vi "Day 9 Task 1 attempt 2.vi"() -> ()   [LabVIEW 2018]
panel:
  out "sum":i32
  out "x+1":i32[][](array[numeric])
  out "subarray":bool[][](array[boolean])
  out "appended array":i32[][](array[numeric])
  out "Array":bool[][](array[boolean])
  out "logical AND":bool
  out "Original Array":i32[][](array[numeric])
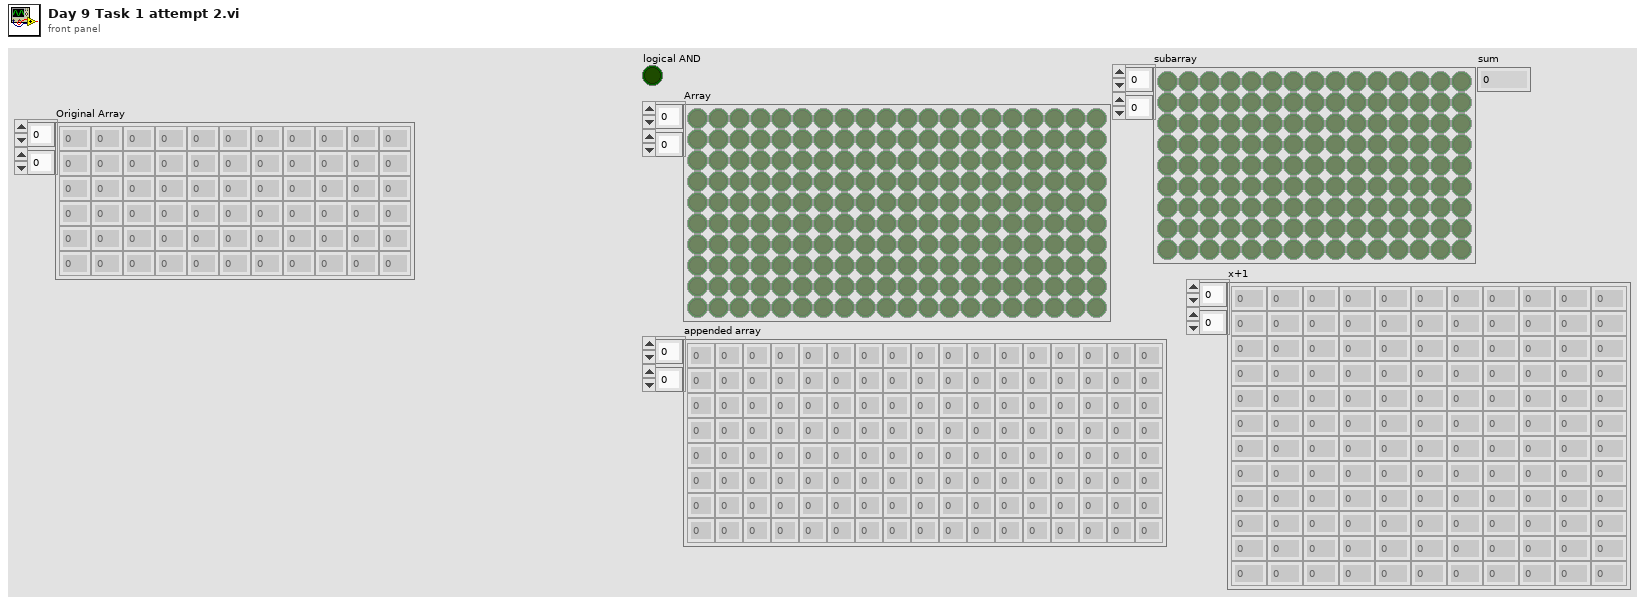
[diagram p1: front panel]
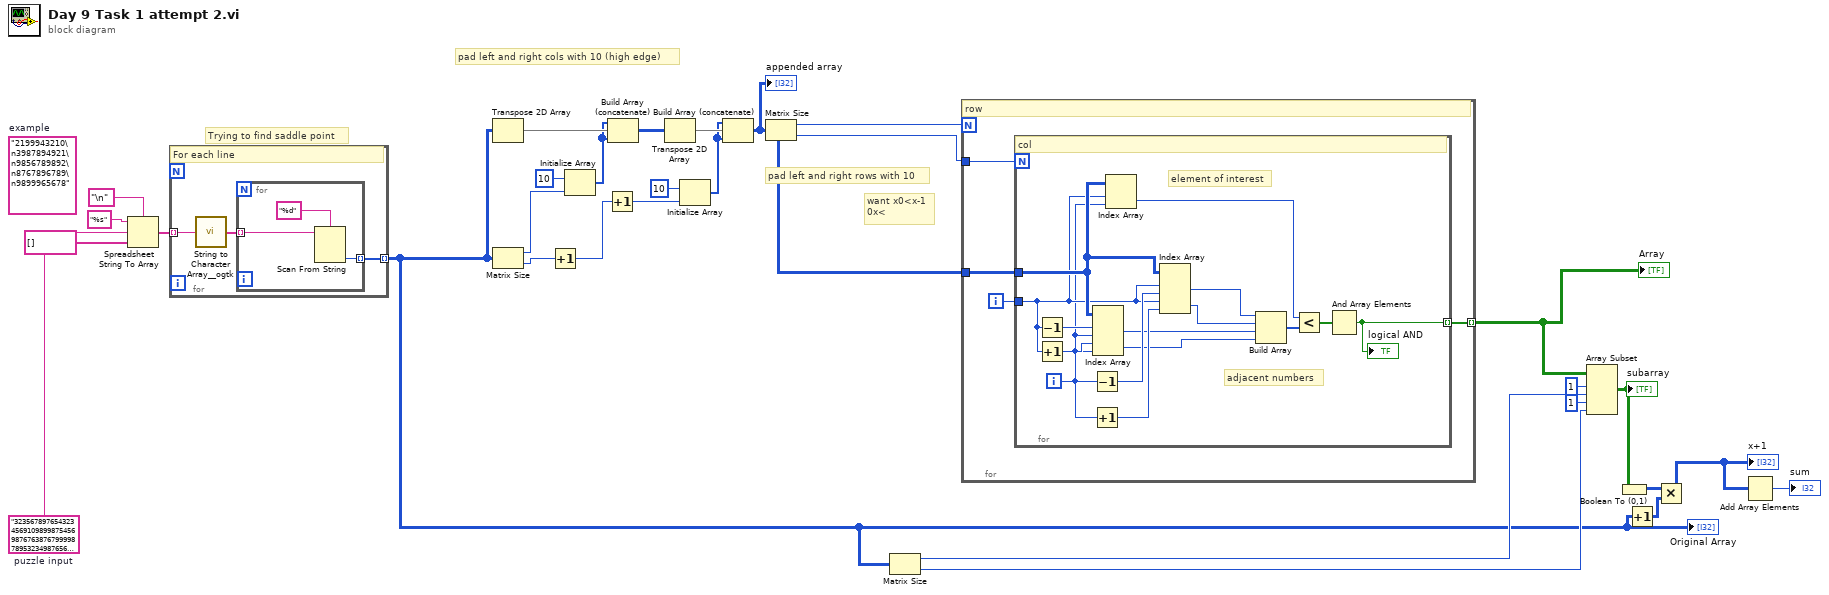
[diagram p0: block diagram]
diagram:
  w1 = "3235678976543234569109899875456987676387679999878953234987656895457998743212347892123999912987632489\n2124899989932145698998789994329876545235567899768995349898546789346987654423656789339889899986541678\n1012567897898756797987678989212985432103458987656789456789435691235998775634987897998776798775430567\n2343489956789987976798899578901299654512578998545899567894326890449899896845898945899655987654321378\n3455697645678999875679965467892398999323456789656798998952018921598799987896789235789544398765435459\n45897894325679877645976543586794978789545789969879879995434594336976898999878921234987321298796..."  # puzzle input
  (unwired) "2199943210\n3987894921\n9856789892\n8767896789\n9899965678"  # example
  # "pad left and right rows with 10"
  # "pad left and right cols with 10 (high edge)"
  # "want x0<x-1\n0x<"
  # "Trying to find saddle point"
  n1 = Spreadsheet String To Array(delimiter (Tab)="\n", format string="%s", spreadsheet string=w1, array type (2D Dbl)=string[] []) -> (array=w28:string[])
  n2 = for {
    tunnel: w28 -> [w33] mode=indexing
    tunnel: [w31] -> w6 mode=indexing
    # "For each line"
    n3 = call <userlib>:"String to Character Array__ogtk.vi"("Input String"=w33) -> ("Character Array"=w32:string[])
    n4 = for {
      tunnel: w32 -> [w36] mode=indexing
      tunnel: [w34] -> w31 mode=indexing
      n5 = Scan From String(format string="%d", input string=w36) -> (output 1=w34:i32)  [unwired: 3 in, 3 out]
    }
  }
  "Original Array" <- w6
  n6 = Transpose 2D Array(2D array=w6) -> (transposed array=w26:i32[][])
  n7 = Matrix Size(0:w6) -> (1:w22:i32, 2:w19:i32)
  n8 = Increment(x=w19) -> (x+1=w16:i32)
  n9 = Initialize Array(10 ("element"), w22) -> (w21:i32[])
  n10 = Increment(x=w16) -> (x+1=w18:i32)
  n11 = Build Array (concatenate)(w21, w26, w21) -> (w25:i32[][])
  n12 = Transpose 2D Array(2D array=w25) -> (transposed array=w20:i32[][])
  n13 = Initialize Array(10 ("number of columns"), w18) -> (w17:i32[])
  n14 = Build Array (concatenate)(w17, w20, w17) -> (w9:i32[][])
  "appended array" <- w9
  n15 = Matrix Size(0:w9) -> (1:w14:i32, 2:w15:i32)
  n16 = Matrix Size(0:w6) -> (1:w11:i32, 2:w10:i32)
  n17 = for {
    N: w14 -> [_]
    tunnel: w9 -> [w40]
    tunnel: w15 -> [w39]
    tunnel: [w37] -> w8 mode=indexing
    i -> [w38]
    # "row"
    n18 = for {
      N: w39 -> [_]
      tunnel: w40 -> [w51]
      tunnel: w38 -> [w48]
      tunnel: [w41] -> w37 mode=indexing
      i -> [w47]
      # "adjacent numbers"
      # "element of interest"
      # "col"
      n19 = Decrement(x=w48) -> (x-1=w50:i32)
      n20 = Increment(x=w48) -> (x+1=w49:i32)
      n21 = Decrement(x=w47) -> (x-1=w55:i32)
      n22 = Increment(x=w47) -> (x+1=w54:i32)
      n23 = Index Array(array=w51, index (row) #1=w50, index (col) #1=w47, index (row) #2=w49, index (col) #2=w47) -> (element #1=w46:i32, element #2=w45:i32)
      n24 = Index Array(array=w51, index (row)=w48, index (col)=w47) -> (element=w44:i32)
      n25 = Index Array(array=w51, index (row) #1=w48, index (col) #1=w55, index (row) #2=w48, index (col) #2=w54) -> (element #1=w53:i32, element #2=w52:i32)
      n26 = Build Array(w53, w52, w46, w45) -> (w43:i32[])
      n27 = Less?(x=w44, y=w43) -> (x < y?=w42:bool[])
      n28 = And Array Elements(Boolean array=w42) -> (logical AND=w41:bool)
      "logical AND" <- w41
    }
  }
  "Array" <- w8
  n29 = Array Subset(array=w8, index (row)=1 ("index"), length (row)=w11, index (col)=1 ("index"), length (col)=w10) -> (w4:bool[][])
  "subarray" <- w4
  n30 = Boolean To (0,1)(Boolean=w4) -> (0, 1=w7:i16[][])
  n31 = Increment(x=w6) -> (x+1=w5:i32[][])
  n32 = Multiply(x=w7, y=w5) -> (x*y=w3:i32[][])
  "x+1" <- w3
  n33 = Add Array Elements(numeric array=w3) -> (sum=→"sum":i32)
